vi "TimeStampToJulianDate.vi"(1 "TimeStamp [UT]":timestamp format="%<%H:%M:%S%6u\n%Y/%m/%d>T") -> (0 "JulianDay":ext format="%.9f")   [LabVIEW 2009]
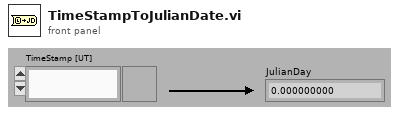
[diagram p1: front panel]
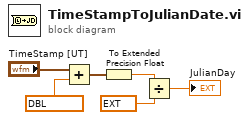
[diagram p0: block diagram]
diagram:
  n1 = Add(x="TimeStamp [UT]", y=ext[unit] 208783915200.0) -> (x+y=w6:timestamp)
  n2 = To Extended Precision Float(1:w6) -> (0:w2:ext)
  n3 = Divide(x=w2, y=ext 86400.0) -> (x/y=→"JulianDay":ext)
